vi "run_experiment_pharmaBot_v0.06.vi"(0 "PhaseX Cluster":T2, 1 "PhaseState":string="A", 2 "current clamp":enum16{"VClamp", "IClamp"}(ring), 3 "time to wait for solution change (min)":dbl=2.5 min=0.0 step=0.01, 4 "valve Time Cluster":T1, 5 "error in":errorcluster, 6 "which manipulator":T4(ring), 7 "common cluster":T6, 8 "Didn't Lift?":bool, 10 "controls array":refnum<vi>[](array[refnum]), 11 "individual controls in":T5, 13 "data in":T3={"daq_ao 1"="Dev1/ao0", "daq_ai 1"="Dev1/ai0", "experiment day folder"=path "D:/DATA/8-27-15 save func testing/test.lvm", "Multiclamp init error"=0, "Multiclamp Handle Out"=0, "sampling rate (Hz)"=10000, "trial name"=""}) -> (12 "control array out":refnum<vi>[](array[refnum]), 14 "protocol waveform":waveform(dbl)[](graph), 15 "protocol response":waveform(dbl)[](graph), 16 "set clamp":enum16{"VClamp", "IClamp"}(ring), 19 "error out":errorcluster)   [LabVIEW 2019]
uses:
  pipette cleaning/pressure box/cleaning_soft/controls/actuator_type.ctl
  pipette cleaning/pressure box/cleaning_soft/controls/actuator_cluster.ctl
  machine_vision/coordinate model vis/transform_properties_actuators.ctl
  machine_vision/controls/transform_cluster_actuator.ctl
  controls/NH_method.ctl
  pipette cleaning/pressure box/cleaning_soft/controls/pressure_box_type.ctl
  pipette cleaning/pressure box/cleaning_soft/controls/pressure_box_control.ctl
  multipatch/controls/multipatch_common_controls_v4.ctl
  controls/memtest_def.ctl
  multipatch/controls/multipatch_individual_controls_v5.ctl
  Controls/Data.ctl
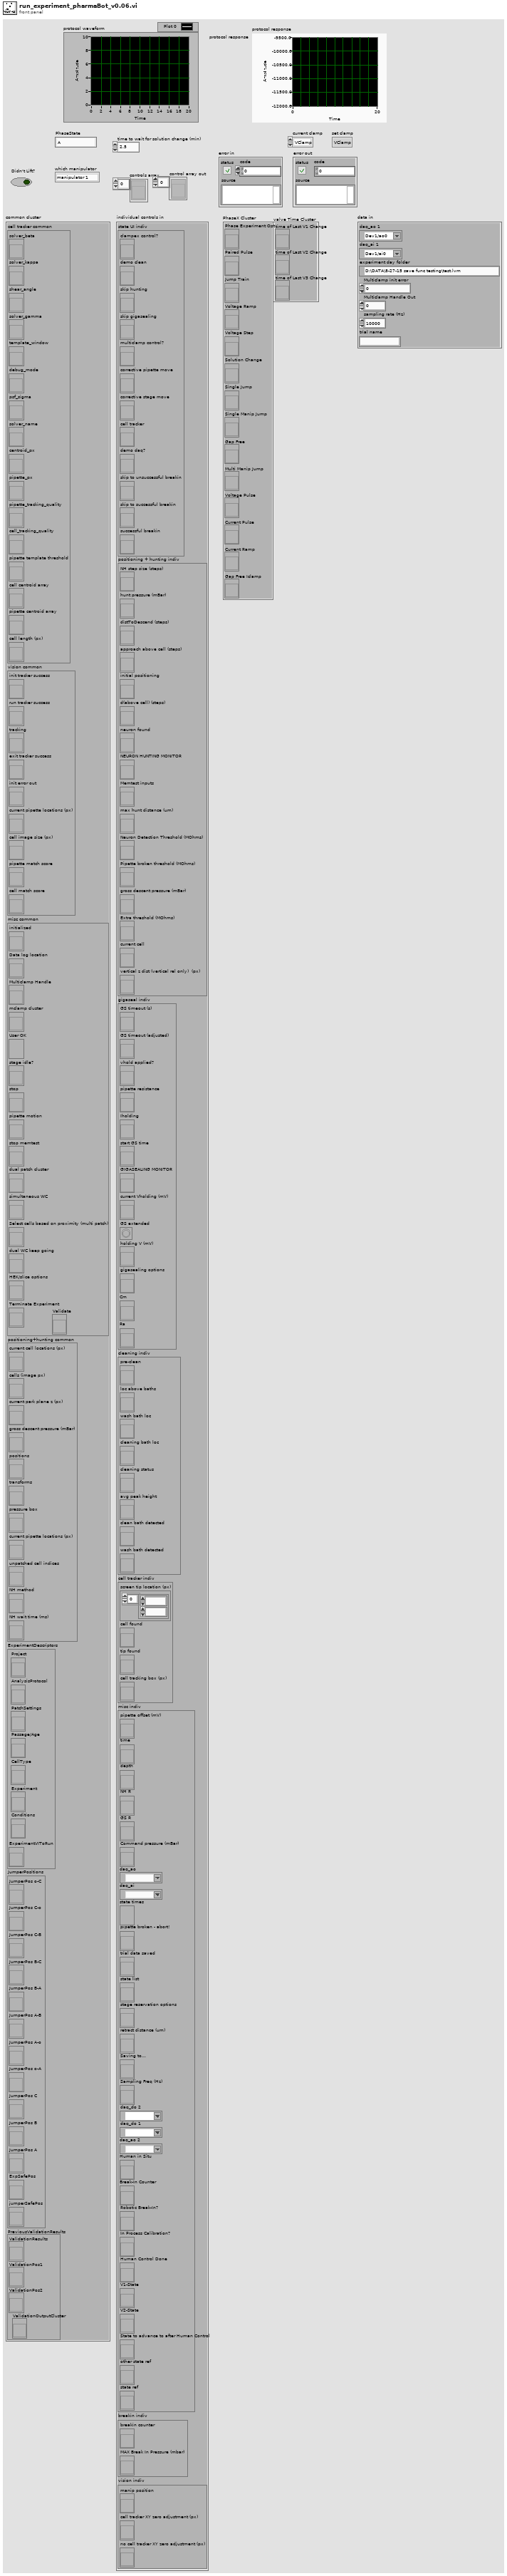
[diagram p1: front panel]
types:
  T1 = cluster{"time of Last V1 Change":refnum<vi>, "time of Last V2 Change":refnum<vi>, "time of Last V3 Change":refnum<vi>}
  T2 = cluster{"Phase Experiment Option":refnum<vi>, "Paired Pulse":refnum<vi>, "Jump Train":refnum<vi>, "Voltage Ramp":refnum<vi>, "Voltage Step":refnum<vi>, "Solution Change":refnum<vi>, "Single Jump":refnum<vi>, "Single Manip Jump":refnum<vi>, "Gap Free":refnum<vi>, "Multi Manip Jump":refnum<vi>, "Voltage Pulse":refnum<vi>, "Current Pulse":refnum<vi>, "Current Ramp":refnum<vi>, "Gap Free Iclamp":refnum<vi>}
  T3 = typedef "Data.ctl" = cluster{"daq_ao 1":tag, "daq_ai 1":tag, "experiment day folder":path, "Multiclamp init error":i32, "Multiclamp Handle Out":u32, "sampling rate (Hz)":i32, "trial name":string}
  T4 = enum16{"manipulator 1", "manipulator 2", "manipulator 3", "manipulator 4"}
  T5 = typedef "multipatch_individual_controls_v5.ctl" = cluster{"state UI indiv":cluster{"clampex control?":refnum<vi>, "demo clean":refnum<vi>, "skip hunting":refnum<vi>, "skip gigasealing":refnum<vi>, "multiclamp control?":refnum<vi>, "corrective pipette move":refnum<vi>, "corrective stage move":refnum<vi>, "cell tracker":refnum<vi>, "demo daq?":refnum<vi>, "skip to unsuccessful breakin":refnum<vi>, "skip to successful breakin":refnum<vi>, "successful breakin":refnum<vi>}, "positioning + hunting indiv":cluster{"NH step size (steps)":refnum<vi>, "hunt pressure (mBar)":refnum<vi>, "distToDescend (steps)":refnum<vi>, "approach above cell (steps)":refnum<vi>, "initial positioning":refnum<vi>, "d(above cell) (steps)":refnum<vi>, "neuron found":refnum<vi>, "NEURON HUNTING MONITOR":refnum<vi>, "Memtest inputs":refnum<vi>, "max hunt distance (um)":refnum<vi>, "Neuron Detection Threshold (MOhms)":refnum<vi>, "Pipette broken threshold (MOhms)":refnum<vi>, "gross descent pressure (mBar)":refnum<vi>, "Extra threshold (MOhms)":refnum<vi>, "current cell":refnum<vi>, "vertical z dist (vertical rel only)  (px)":refnum<vi>}, "gigaseal indiv":cluster{"GS timeout (s)":refnum<vi>, "GS timeout (adjusted)":refnum<vi>, "vhold applied?":refnum<vi>, "pipette resistance":refnum<vi>, "Iholding":refnum<vi>, "start GS time":refnum<vi>, "GIGASEALING MONITOR":refnum<vi>, "current Vholding (mV)":refnum<vi>, "GS extended":refnum<vi>, "holding V (mV)":refnum<vi>, "gigasealing options":refnum<vi>, "Cm":refnum<vi>, "Ra ":refnum<vi>}, "cleaning indiv":cluster{"pre-clean":refnum<vi>, "loc above baths":refnum<vi>, "wash bath loc":refnum<vi>, "cleaning bath loc":refnum<vi>, "cleaning status":refnum<vi>, "avg peak height":refnum<vi>, "clean bath detected":refnum<vi>, "wash bath detected":refnum<vi>}, "cell tracker indiv":cluster{"screen tip location (px)":refnum<vi>, "cell found":refnum<vi>, "tip found":refnum<vi>, "cell tracking box (px)":refnum<vi>}, "misc indiv":cluster{"pipette offset (mV)":refnum<vi>, "time":refnum<vi>, "depth":refnum<vi>, "NH R":refnum<vi>, "GS R":refnum<vi>, "Command pressure (mBar)":refnum<vi>, "daq_ao":tag, "daq_ai":tag, "state times":refnum<vi>, "pipette broken - abort!":refnum<vi>, "trial data saved":refnum<vi>, "state list":refnum<vi>, "stage reservation options":refnum<vi>, "retract distance (um)":refnum<vi>, "Saving to...":refnum<vi>, "Sampling Freq (Hz)":refnum<vi>, "daq_do 2":tag, "daq_do 1":tag, "daq_ao 2":tag, "Human in Situ":refnum<vi>, "Break-In Counter":refnum<vi>, "Robotic Break-In?":refnum<vi>, "In Process Calibration?":refnum<vi>, "Human Control Done":refnum<vi>, "V1-State":refnum<vi>, "V2-State":refnum<vi>, "State to advance to after Human Control":refnum<vi>, "other state ref":refnum<vi>, "state ref":refnum<vi>}, "breakin indiv":cluster{"breakin counter":refnum<vi>, "MAX Break In Pressure (mbar)":refnum<vi>}, "vision indiv":cluster{"manip position":refnum<vi>, "cell tracker XY zero adjustment (px)":refnum<vi>, "no cell tracker XY zero adjustment (px)":refnum<vi>}}
  T6 = typedef "multipatch_common_controls_v4.ctl" = cluster{"cell tracker common":cluster{"solver_beta":refnum<vi>, "solver_kappa":refnum<vi>, "shear_angle":refnum<vi>, "solver_gamma":refnum<vi>, "template_window":refnum<vi>, "debug_mode":refnum<vi>, "psf_sigma":refnum<vi>, "solver_name":refnum<vi>, "centroid_px":refnum<vi>, "pipette_px":refnum<vi>, "pipette_tracking_quality":refnum<vi>, "cell_tracking_quality":refnum<vi>, "pipette template threshold":refnum<vi>, "cell centroid array":refnum<vi>, "pipette centroid array":refnum<vi>, "cell length (px)":refnum<vi>}, "vision common":cluster{"init tracker success":refnum<vi>, "run tracker success":refnum<vi>, "tracking":refnum<vi>, "exit tracker success":refnum<vi>, "init error out":refnum<vi>, "current pipette locations (px)":refnum<vi>, "cell image size (px)":refnum<vi>, "pipette match score":refnum<vi>, "cell match score":refnum<vi>}, "misc common":cluster{"initialized":refnum<vi>, "Data log location":refnum<vi>, "Multiclamp Handle":refnum<vi>, "mclamp cluster":refnum<vi>, "User OK":refnum<vi>, "stage idle?":refnum<vi>, "stop":refnum<vi>, "pipette motion":refnum<vi>, "stop memtest":refnum<vi>, "dual patch cluster":refnum<vi>, "simultaneous WC":refnum<vi>, "Select cells based on proximity (multi patch)":refnum<vi>, "dual WC keep going":refnum<vi>, "HEK/slice options":refnum<vi>, "Terminate Experiment":refnum<vi>, "Validate":refnum<vi>}, "positioning+hunting common":cluster{"current cell locations (px)":refnum<vi>, "cells (image px)":refnum<vi>, "current park plane z (px)":refnum<vi>, "gross descent pressure (mBar)":refnum<vi>, "positions":refnum<vi>, "transforms":refnum<vi>, "pressure box":refnum<vi>, "current pipette locations (px)":refnum<vi>, "unpatched cell indices":refnum<vi>, "NH method":refnum<vi>, "NH wait time (ms)":refnum<vi>}, "ExperimentDescriptors":cluster{"Project":refnum<vi>, "AnalysisProtocol":refnum<vi>, "PatchSettings":refnum<vi>, "Passage/Age":refnum<vi>, "CellType":refnum<vi>, "Experiment":refnum<vi>, "Conditions":refnum<vi>, "ExperimentVIToRun":refnum<vi>}, "JumperPositions":cluster{"JumperPos o-C":refnum<vi>, "JumperPos C-o":refnum<vi>, "JumperPos C-B":refnum<vi>, "JumperPos B-C":refnum<vi>, "JumperPos B-A":refnum<vi>, "JumperPos A-B":refnum<vi>, "JumperPos A-o":refnum<vi>, "JumperPos o-A":refnum<vi>, "JumperPos C":refnum<vi>, "JumperPos B":refnum<vi>, "JumperPos A":refnum<vi>, "ExpSafePos":refnum<vi>, "jumperSafePos":refnum<vi>}, "PreviousValidationResults":cluster{"ValidationResults":refnum<vi>, "ValidationPos1":refnum<vi>, "ValidationPos2":refnum<vi>, "ValidationOutputCluster":refnum<vi>}}
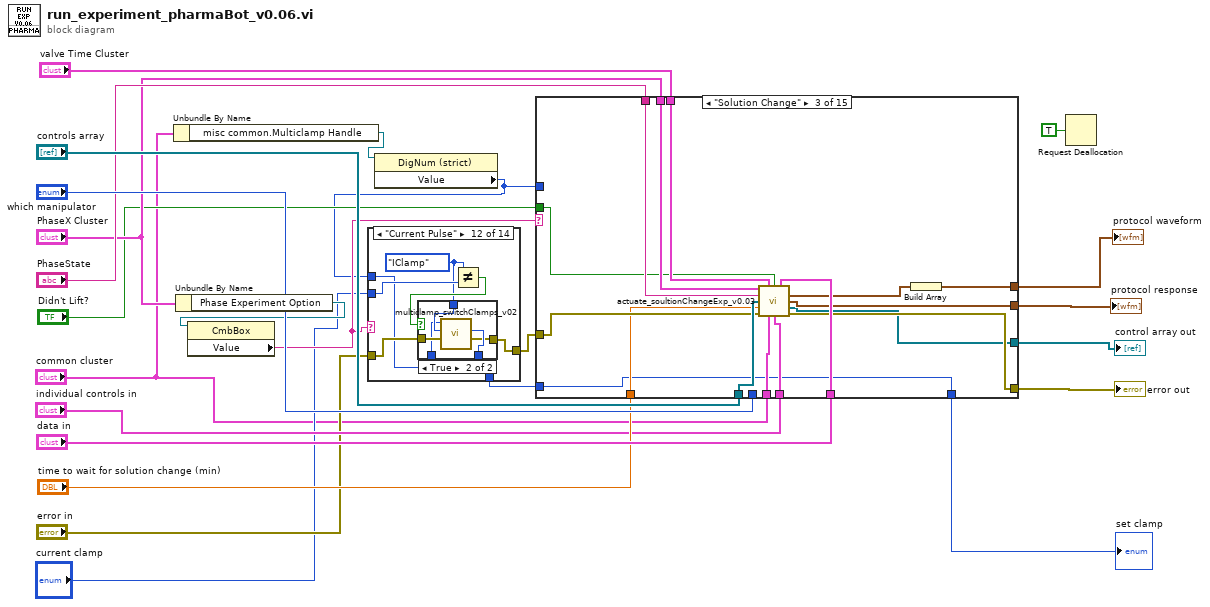
[diagram p0: block diagram]
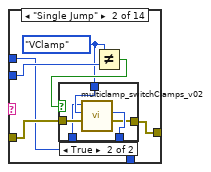
[diagram p3: hidden frame]
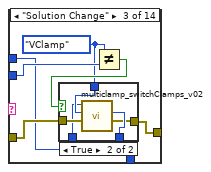
[diagram p5: hidden frame]
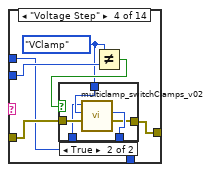
[diagram p7: hidden frame]
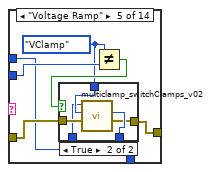
[diagram p9: hidden frame]
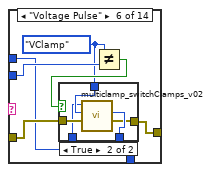
[diagram p11: hidden frame]
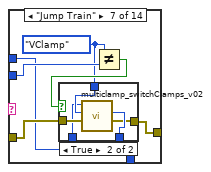
[diagram p13: hidden frame]
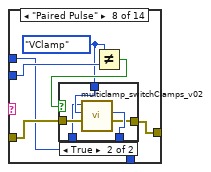
[diagram p15: hidden frame]
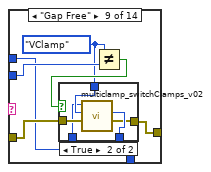
[diagram p17: hidden frame]
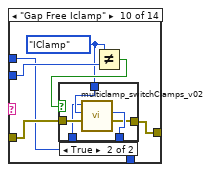
[diagram p19: hidden frame]
diagram:
  n1 = Unbundle By Name("common cluster") -> ("misc common.Multiclamp Handle"=w4:refnum<vi>)
  n2 = Unbundle By Name("PhaseX Cluster") -> ("Phase Experiment Option"=w20:refnum<vi>)
  n3 = property class="CmbBox"(reference=w20) -> ("Value"=w7:string)  [unwired: 1 in, 2 out]
  n4 = property class="DigNum (strict)"(reference=w4) -> ("Value"=w1:u32)  [unwired: 1 in, 2 out]
  n5 = case shown="\"Current Pulse\"" w7 {
    tunnel: [w25 w33 w47 w61 w75 w89 w103 w117 w131 w145 w159 w173 w187 w201] -> w3
    tunnel: "error in" -> [w26 w32 w46 w60 w74 w88 w102 w116 w130 w144 w158 w172 w186 w200]
    tunnel: [w26 w31 w45 w59 w73 w87 w101 w115 w129 w143 w157 w171 w185 w199] -> w8
    tunnel: "current clamp" -> [w25 w30 w44 w58 w72 w86 w100 w114 w128 w142 w156 w170 w184 w198]
    tunnel: w1 -> [_ w27 w41 w55 w69 w83 w97 w111 w125 w139 w153 w167 w181 w195]
    frame "False", Default {
    }
    frame "Single Jump" {
      w28 = enum16{"VClamp", "IClamp"}."VClamp" ("current clamp mode")
      n6 = Not Equal?(x=w28, y=w30) -> (x != y?=w29:bool)
      n7 = case shown="True" w29 {
        tunnel: [w35 w40] -> w33
        tunnel: w32 -> [w34 w39]
        tunnel: [w34 w38] -> w31
        tunnel: w28 -> [w35 w37]
        tunnel: w27 -> [_ w36]
        frame False {
        }
        frame True {
          n8 = call "multiclamp_switchClamps_v02.vi"("error in (no error)"=w39, "which clamp"=w37, "Multiclamp Handle in"=w36) -> ("error out"=w38:errorcluster, "current clamp mode"=w40:enum16{"VClamp", "IClamp"})  [unwired: 7 in]
        }
      }
    }
    frame "Solution Change" {
      w42 = enum16{"VClamp", "IClamp"}."VClamp" ("current clamp mode")
      n9 = Not Equal?(x=w42, y=w44) -> (x != y?=w43:bool)
      n10 = case shown="True" w43 {
        tunnel: [w49 w54] -> w47
        tunnel: w46 -> [w48 w53]
        tunnel: [w48 w52] -> w45
        tunnel: w42 -> [w49 w51]
        tunnel: w41 -> [_ w50]
        frame False {
        }
        frame True {
          n11 = call "multiclamp_switchClamps_v02.vi"("error in (no error)"=w53, "which clamp"=w51, "Multiclamp Handle in"=w50) -> ("error out"=w52:errorcluster, "current clamp mode"=w54:enum16{"VClamp", "IClamp"})  [unwired: 7 in]
        }
      }
    }
    frame "Voltage Step" {
      w56 = enum16{"VClamp", "IClamp"}."VClamp" ("current clamp mode")
      n12 = Not Equal?(x=w56, y=w58) -> (x != y?=w57:bool)
      n13 = case shown="True" w57 {
        tunnel: [w63 w68] -> w61
        tunnel: w60 -> [w62 w67]
        tunnel: [w62 w66] -> w59
        tunnel: w56 -> [w63 w65]
        tunnel: w55 -> [_ w64]
        frame False {
        }
        frame True {
          n14 = call "multiclamp_switchClamps_v02.vi"("error in (no error)"=w67, "which clamp"=w65, "Multiclamp Handle in"=w64) -> ("error out"=w66:errorcluster, "current clamp mode"=w68:enum16{"VClamp", "IClamp"})  [unwired: 7 in]
        }
      }
    }
    frame "Voltage Ramp" {
      w70 = enum16{"VClamp", "IClamp"}."VClamp" ("current clamp mode")
      n15 = Not Equal?(x=w70, y=w72) -> (x != y?=w71:bool)
      n16 = case shown="True" w71 {
        tunnel: [w77 w82] -> w75
        tunnel: w74 -> [w76 w81]
        tunnel: [w76 w80] -> w73
        tunnel: w70 -> [w77 w79]
        tunnel: w69 -> [_ w78]
        frame False {
        }
        frame True {
          n17 = call "multiclamp_switchClamps_v02.vi"("error in (no error)"=w81, "which clamp"=w79, "Multiclamp Handle in"=w78) -> ("error out"=w80:errorcluster, "current clamp mode"=w82:enum16{"VClamp", "IClamp"})  [unwired: 7 in]
        }
      }
    }
    frame "Voltage Pulse" {
      w84 = enum16{"VClamp", "IClamp"}."VClamp" ("current clamp mode")
      n18 = Not Equal?(x=w84, y=w86) -> (x != y?=w85:bool)
      n19 = case shown="True" w85 {
        tunnel: [w91 w96] -> w89
        tunnel: w88 -> [w90 w95]
        tunnel: [w90 w94] -> w87
        tunnel: w84 -> [w91 w93]
        tunnel: w83 -> [_ w92]
        frame False {
        }
        frame True {
          n20 = call "multiclamp_switchClamps_v02.vi"("error in (no error)"=w95, "which clamp"=w93, "Multiclamp Handle in"=w92) -> ("error out"=w94:errorcluster, "current clamp mode"=w96:enum16{"VClamp", "IClamp"})  [unwired: 7 in]
        }
      }
    }
    frame "Jump Train" {
      w98 = enum16{"VClamp", "IClamp"}."VClamp" ("current clamp mode")
      n21 = Not Equal?(x=w98, y=w100) -> (x != y?=w99:bool)
      n22 = case shown="True" w99 {
        tunnel: [w105 w110] -> w103
        tunnel: w102 -> [w104 w109]
        tunnel: [w104 w108] -> w101
        tunnel: w98 -> [w105 w107]
        tunnel: w97 -> [_ w106]
        frame False {
        }
        frame True {
          n23 = call "multiclamp_switchClamps_v02.vi"("error in (no error)"=w109, "which clamp"=w107, "Multiclamp Handle in"=w106) -> ("error out"=w108:errorcluster, "current clamp mode"=w110:enum16{"VClamp", "IClamp"})  [unwired: 7 in]
        }
      }
    }
    frame "Paired Pulse" {
      w112 = enum16{"VClamp", "IClamp"}."VClamp" ("current clamp mode")
      n24 = Not Equal?(x=w112, y=w114) -> (x != y?=w113:bool)
      n25 = case shown="True" w113 {
        tunnel: [w119 w124] -> w117
        tunnel: w116 -> [w118 w123]
        tunnel: [w118 w122] -> w115
        tunnel: w112 -> [w119 w121]
        tunnel: w111 -> [_ w120]
        frame False {
        }
        frame True {
          n26 = call "multiclamp_switchClamps_v02.vi"("error in (no error)"=w123, "which clamp"=w121, "Multiclamp Handle in"=w120) -> ("error out"=w122:errorcluster, "current clamp mode"=w124:enum16{"VClamp", "IClamp"})  [unwired: 7 in]
        }
      }
    }
    frame "Gap Free" {
      w126 = enum16{"VClamp", "IClamp"}."VClamp" ("current clamp mode")
      n27 = Not Equal?(x=w126, y=w128) -> (x != y?=w127:bool)
      n28 = case shown="True" w127 {
        tunnel: [w133 w138] -> w131
        tunnel: w130 -> [w132 w137]
        tunnel: [w132 w136] -> w129
        tunnel: w126 -> [w133 w135]
        tunnel: w125 -> [_ w134]
        frame False {
        }
        frame True {
          n29 = call "multiclamp_switchClamps_v02.vi"("error in (no error)"=w137, "which clamp"=w135, "Multiclamp Handle in"=w134) -> ("error out"=w136:errorcluster, "current clamp mode"=w138:enum16{"VClamp", "IClamp"})  [unwired: 7 in]
        }
      }
    }
    frame "Gap Free Iclamp" {
      w140 = enum16{"VClamp", "IClamp"}."IClamp" ("current clamp mode")
      n30 = Not Equal?(x=w140, y=w142) -> (x != y?=w141:bool)
      n31 = case shown="True" w141 {
        tunnel: [w147 w152] -> w145
        tunnel: w144 -> [w146 w151]
        tunnel: [w146 w150] -> w143
        tunnel: w140 -> [w147 w149]
        tunnel: w139 -> [_ w148]
        frame False {
        }
        frame True {
          n32 = call "multiclamp_switchClamps_v02.vi"("error in (no error)"=w151, "which clamp"=w149, "Multiclamp Handle in"=w148) -> ("error out"=w150:errorcluster, "current clamp mode"=w152:enum16{"VClamp", "IClamp"})  [unwired: 7 in]
        }
      }
    }
    frame "Current Ramp" {
      w154 = enum16{"VClamp", "IClamp"}."IClamp" ("current clamp mode")
      n33 = Not Equal?(x=w154, y=w156) -> (x != y?=w155:bool)
      n34 = case shown="True" w155 {
        tunnel: [w161 w166] -> w159
        tunnel: w158 -> [w160 w165]
        tunnel: [w160 w164] -> w157
        tunnel: w154 -> [w161 w163]
        tunnel: w153 -> [_ w162]
        frame False {
        }
        frame True {
          n35 = call "multiclamp_switchClamps_v02.vi"("error in (no error)"=w165, "which clamp"=w163, "Multiclamp Handle in"=w162) -> ("error out"=w164:errorcluster, "current clamp mode"=w166:enum16{"VClamp", "IClamp"})  [unwired: 7 in]
        }
      }
    }
    frame "Current Pulse" {
      w168 = enum16{"VClamp", "IClamp"}."IClamp" ("current clamp mode")
      n36 = Not Equal?(x=w168, y=w170) -> (x != y?=w169:bool)
      n37 = case shown="True" w169 {
        tunnel: [w175 w180] -> w173
        tunnel: w172 -> [w174 w179]
        tunnel: [w174 w178] -> w171
        tunnel: w168 -> [w175 w177]
        tunnel: w167 -> [_ w176]
        frame False {
        }
        frame True {
          n38 = call "multiclamp_switchClamps_v02.vi"("error in (no error)"=w179, "which clamp"=w177, "Multiclamp Handle in"=w176) -> ("error out"=w178:errorcluster, "current clamp mode"=w180:enum16{"VClamp", "IClamp"})  [unwired: 7 in]
        }
      }
    }
    frame "Multi M. Jump" {
      w182 = enum16{"VClamp", "IClamp"}."VClamp" ("current clamp mode")
      n39 = Not Equal?(x=w182, y=w184) -> (x != y?=w183:bool)
      n40 = case shown="True" w183 {
        tunnel: [w189 w194] -> w187
        tunnel: w186 -> [w188 w193]
        tunnel: [w188 w192] -> w185
        tunnel: w182 -> [w189 w191]
        tunnel: w181 -> [_ w190]
        frame False {
        }
        frame True {
          n41 = call "multiclamp_switchClamps_v02.vi"("error in (no error)"=w193, "which clamp"=w191, "Multiclamp Handle in"=w190) -> ("error out"=w192:errorcluster, "current clamp mode"=w194:enum16{"VClamp", "IClamp"})  [unwired: 7 in]
        }
      }
    }
    frame "Single Manip Jump" {
      w196 = enum16{"VClamp", "IClamp"}."VClamp" ("current clamp mode")
      n42 = Not Equal?(x=w196, y=w198) -> (x != y?=w197:bool)
      n43 = case shown="True" w197 {
        tunnel: [w203 w208] -> w201
        tunnel: w200 -> [w202 w207]
        tunnel: [w202 w206] -> w199
        tunnel: w196 -> [w203 w205]
        tunnel: w195 -> [_ w204]
        frame False {
        }
        frame True {
          n44 = call "multiclamp_switchClamps_v02.vi"("error in (no error)"=w207, "which clamp"=w205, "Multiclamp Handle in"=w204) -> ("error out"=w206:errorcluster, "current clamp mode"=w208:enum16{"VClamp", "IClamp"})  [unwired: 7 in]
        }
      }
    }
  }
  n45 = case shown="\"Solution Change\"" w7 {
    tunnel: "PhaseX Cluster" -> [_ w230 w241 w260 w275 w293 w308 w326 w342 w356 w369 w387 w404 w420 _]
    tunnel: w8 -> [w214 w228 w240 w251 w269 w287 w302 w320 w338 w357 w362 w380 w400 w418 w426]
    tunnel: [w214 w224 w239 w254 w268 w278 w301 w311 w337 w357 w361 w374 w399 w414 w426] -> w14
    tunnel: "data in" -> [_ w225 w246 w258 w264 w283 w297 w316 w336 w352 w370 w388 w398 w415 _]
    tunnel: "individual controls in" -> [_ w226 w245 w249 w265 w284 w298 w317 w332 w345 w371 w389 w396 w416 _]
    tunnel: "common cluster" -> [_ w227 w244 w250 w266 w285 w299 w318 w331 w346 w372 w390 w397 w417 _]
    tunnel: "which manipulator" -> [_ _ _ _ _ _ _ _ _ _ _ _ _ _ _]
    tunnel: "controls array" -> [w213 w229 w243 w253 w273 w291 w306 w324 w340 w348 w365 w383 w402 w419 w425]
    tunnel: "PhaseState" -> [_ w223 w242 w259 w274 w292 w307 w325 w341 w355 w368 w386 w403 w413 _]
    tunnel: [waveform(dbl)[] [] ("protcol response") w222 w238 w256 w270 w288 w303 w321 w334 w350 w360 w379 w393 w412 waveform(dbl)[] [] ("protcol response")] -> w13
    tunnel: [w210 w216 w232 w257 w271 w289 w304 w322 w330 w351 waveform(dbl)[] [] ("protocol waveform") waveform(dbl)[] [] ("protocol waveform") w392 w407 w422] -> w12
    tunnel: [w213 w220 w236 w255 w272 w290 w305 w323 w333 w349 w364 w382 w395 w410 w425] -> w11
    tunnel: "time to wait for solution change (min)" -> [_ w219 w235 w252 w267 w286 w300 w319 w339 w347 w363 w381 w401 w409 _]
    tunnel: "valve Time Cluster" -> [_ w218 w234 w261 w276 w294 w309 w327 w343 w354 w367 w385 w405 w408 _]
    tunnel: "Didn't Lift?" -> [_ w217 w233 w248 w263 w282 w296 w315 w329 w353 w366 w384 _ _ _]
    tunnel: w3 -> [w209 w215 w231 w247 w262 _ w295 _ w328 w344 w358 _ w391 w406 w421]
    tunnel: [w209 w215 w231 w247 w262 w277 w295 w310 w328 w344 w358 w373 w391 w406 w421] -> w2
    tunnel: w1 -> [_ _ _ _ _ w281 _ w314 _ _ _ w376 _ _ _]
    frame "False", Default {
      n46 = Build Array(waveform(dbl) {"t0"=timestamp(0 s since 1904-01-01), "dt"=1.0, "Y"=[]} ("jumptestMonitor")) -> (w210:waveform(dbl)[])
    }
    frame "Single Jump" {
      n47 = call "actuate_singleJumpExp_v0.04.vi"("Phase Cluster"=w230, "valve Time Cluster"=w218, "Didn't Lift?"=w217, "data in"=w225, "PhaseLetter"=w223, "controls array in"=w229, "time to wait for solution change (min)"=w219, "error in"=w228, "common cluster"=w227, "individual controls in"=w226) -> ("protocol waveform"=w221:waveform(dbl), "jumptestMonitor"=w222:waveform(dbl)[], "control array out"=w220:refnum<vi>[], "error out"=w224:errorcluster)  [unwired: 2 out]
      n48 = Build Array(w221) -> (w216:waveform(dbl)[])
    }
    frame "Solution Change" {
      n49 = call "actuate_soultionChangeExp_v0.03.vi"("Phase Cluster"=w241, "valve Time Cluster"=w234, "Didn't Lift?"=w233, "data in"=w246, "PhaseLetter"=w242, "controls array in"=w243, "time to wait for solution change (min)"=w235, "error in"=w240, "common cluster"=w244, "individual controls in"=w245) -> ("protocol waveform"=w237:waveform(dbl), "jumptestMonitor"=w238:waveform(dbl)[], "control array out"=w236:refnum<vi>[], "error out"=w239:errorcluster)  [unwired: 2 out]
      n50 = Build Array(w237) -> (w232:waveform(dbl)[])
    }
    frame "Voltage Step" {
      n51 = call "actuate_voltageStepExp_v0.05.vi"("Phase Cluster"=w260, "valve Time Cluster"=w261, "Didn't Lift?"=w248, "data in"=w258, "PhaseLetter"=w259, "controls array in"=w253, "time to wait for solution change (min)"=w252, "error in"=w251, "common cluster"=w250, "individual controls in"=w249) -> ("protocol waveform"=w257:waveform(dbl)[], "jumptestMonitor"=w256:waveform(dbl)[], "control array out"=w255:refnum<vi>[], "error out"=w254:errorcluster)  [unwired: 2 out]
    }
    frame "Voltage Ramp" {
      n52 = call "actuate_voltageRampExp_v0.05.vi"("Phase Cluster"=w275, "valve Time Cluster"=w276, "Didn't Lift?"=w263, "data in"=w264, "PhaseLetter"=w274, "controls array in"=w273, "time to wait for solution change (min)"=w267, "error in"=w269, "common cluster"=w266, "individual controls in"=w265) -> ("protocol waveform"=w271:waveform(dbl)[], "jumptestMonitor"=w270:waveform(dbl)[], "control array out"=w272:refnum<vi>[], "error out"=w268:errorcluster)  [unwired: 2 out]
    }
    frame "Current Ramp" {
      n53 = call "actuate_currentRampExp_v0.05.vi"("Phase Cluster"=w293, "valve Time Cluster"=w294, "Didn't Lift?"=w282, "data in"=w283, "PhaseLetter"=w292, "controls array in"=w291, "time to wait for solution change (min)"=w286, "error in"=w287, "common cluster"=w285, "individual controls in"=w284) -> ("protocol waveform"=w289:waveform(dbl)[], "jumptestMonitor"=w288:waveform(dbl)[], "control array out"=w290:refnum<vi>[], "error out"=w279:errorcluster)  [unwired: 2 out]
      n54 = call "multiclamp_switchClamps_v02.vi"("error in (no error)"=w279, "which clamp"=enum16{"VClamp", "IClamp"}."VClamp", "Multiclamp Handle in"=w281) -> ("error out"=w278:errorcluster, "current clamp mode"=w277:enum16{"VClamp", "IClamp"})  [unwired: 7 in]
    }
    frame "Voltage Pulse" {
      n55 = call "actuate_voltagePulseExp_v0.05.vi"("Phase Cluster"=w308, "valve Time Cluster"=w309, "Didn't Lift?"=w296, "data in"=w297, "PhaseLetter"=w307, "controls array in"=w306, "time to wait for solution change (min)"=w300, "error in"=w302, "common cluster"=w299, "individual controls in"=w298) -> ("protocol waveform"=w304:waveform(dbl)[], "jumptestMonitor"=w303:waveform(dbl)[], "control array out"=w305:refnum<vi>[], "error out"=w301:errorcluster)  [unwired: 2 out]
    }
    frame "Current Pulse" {
      n56 = call "actuate_currentPulseExp_v0.05.vi"("Phase Cluster"=w326, "valve Time Cluster"=w327, "Didn't Lift?"=w315, "data in"=w316, "PhaseLetter"=w325, "controls array in"=w324, "time to wait for solution change (min)"=w319, "error in"=w320, "common cluster"=w318, "individual controls in"=w317) -> ("protocol waveform"=w322:waveform(dbl)[], "jumptestMonitor"=w321:waveform(dbl)[], "control array out"=w323:refnum<vi>[], "error out"=w312:errorcluster)  [unwired: 2 out]
      n57 = call "multiclamp_switchClamps_v02.vi"("error in (no error)"=w312, "which clamp"=enum16{"VClamp", "IClamp"}."VClamp", "Multiclamp Handle in"=w314) -> ("error out"=w311:errorcluster, "current clamp mode"=w310:enum16{"VClamp", "IClamp"})  [unwired: 7 in]
    }
    frame "Jump Train" {
      n58 = call "actuate_JumpTrainExp_v0.04.vi"("Phase Cluster"=w342, "valve Time Cluster"=w343, "Didn't Lift?"=w329, "data in"=w336, "PhaseLetter"=w341, "controls array in"=w340, "time to wait for solution change (min)"=w339, "error in"=w338, "common cluster"=w331, "individual controls in"=w332) -> ("protocol waveform"=w335:waveform(dbl), "jumptestMonitor"=w334:waveform(dbl)[], "control array out"=w333:refnum<vi>[], "error out"=w337:errorcluster)  [unwired: 2 out]
      n59 = Build Array(w335) -> (w330:waveform(dbl)[])
    }
    frame "Paired Pulse" {
      n60 = call "actuate_PairedPulseExp_v0.04.vi"("Phase Cluster"=w356, "valve Time Cluster"=w354, "Didn't Lift?"=w353, "data in"=w352, "PhaseLetter"=w355, "controls array in"=w348, "time to wait for solution change (min)"=w347, "common cluster"=w346, "individual controls in"=w345) -> ("protocol waveform"=w351:waveform(dbl)[], "jumptestMonitor"=w350:waveform(dbl)[], "control array out"=w349:refnum<vi>[])  [unwired: 1 in, 3 out]
    }
    frame "Gap Free" {
      n61 = call "actuate_gapFreeExp_v0.04.vi"("Phase Cluster"=w369, "valve Time Cluster"=w367, "Didn't Lift?"=w366, "data in"=w370, "PhaseLetter"=w368, "controls array in"=w365, "time to wait for solution change (min)"=w363, "error in"=w362, "common cluster"=w372, "individual controls in"=w371) -> ("jumptestMonitor"=w360:waveform(dbl)[], "control array out"=w364:refnum<vi>[], "error out"=w361:errorcluster)  [unwired: 1 in, 2 out]
    }
    frame "Gap Free Iclamp" {
      n62 = call "actuate_gapFreeIclampExp_v0.04.vi"("Phase Cluster"=w387, "valve Time Cluster"=w385, "Didn't Lift?"=w384, "data in"=w388, "PhaseLetter"=w386, "controls array in"=w383, "time to wait for solution change (min)"=w381, "error in"=w380, "common cluster"=w390, "individual controls in"=w389) -> ("jumptestMonitor"=w379:waveform(dbl)[], "control array out"=w382:refnum<vi>[], "error out"=w375:errorcluster)  [unwired: 1 in, 2 out]
      n63 = call "multiclamp_switchClamps_v02.vi"("error in (no error)"=w375, "which clamp"=enum16{"VClamp", "IClamp"}."VClamp", "Multiclamp Handle in"=w376) -> ("error out"=w374:errorcluster, "current clamp mode"=w373:enum16{"VClamp", "IClamp"})  [unwired: 7 in]
    }
    frame "Multi M. Jump" {
      n64 = call "actuate_multiManipJumpExp_v0.02.vi"("Phase Cluster"=w404, "valve Time Cluster"=w405, "data in"=w398, "PhaseLetter"=w403, "controls array in"=w402, "time to wait for solution change (min)"=w401, "error in"=w400, "common cluster"=w397, "individual controls in"=w396) -> ("protocol waveform"=w394:waveform(dbl), "protcol response"=w393:waveform(dbl)[], "control array out"=w395:refnum<vi>[], "error out"=w399:errorcluster)  [unwired: 1 in, 2 out]
      n65 = Build Array(w394) -> (w392:waveform(dbl)[])
    }
    frame "Single Manip Jump" {
      n66 = call "actuate_singleManipJumpExp_v0.03.vi"("Phase Cluster"=w420, "valve Time Cluster"=w408, "data in"=w415, "PhaseLetter"=w413, "controls array in"=w419, "time to wait for solution change (min)"=w409, "error in"=w418, "common cluster"=w417, "individual controls in"=w416) -> ("protocol waveform"=w411:waveform(dbl), "protcol response"=w412:waveform(dbl)[], "control array out"=w410:refnum<vi>[], "error out"=w414:errorcluster)  [unwired: 1 in, 2 out]
      n67 = Build Array(w411) -> (w407:waveform(dbl)[])
    }
    frame "none" {
      n68 = Build Array(waveform(dbl) {"t0"=timestamp(0 s since 1904-01-01), "dt"=1.0, "Y"=[]} ("jumptestMonitor")) -> (w422:waveform(dbl)[])
    }
  }
  "error out" <- w14
  "protocol response" <- w13
  "protocol waveform" <- w12
  "control array out" <- w11
  "set clamp" <- w2
  n69 = Request Deallocation(TRUE ("flag")) -> ()
